vi "Test Pass if in Map.vi"(8 "error in (no error)":errorcluster, 11 "Dummy In":refnum<class "Example Test Case.lvclass">) -> (0 "error out":errorcluster, 3 "Dummy Out":refnum<class "Example Test Case.lvclass">)   [LabVIEW 2020, in "Example Test Case.lvclass"]
doc: "Failing test"
uses:
  Example Test Case.lvclass
  C:/git/astemes-lunit/source/API/LUnit Test Case/LUnit Test Case.lvclass
  API/LUnit Test Case/LUnit Test Case.lvclass/LUnit Test Case.ctl
  f7599997-06c6-4163-a399-60519fa8dddf.vi
  API/LUnit Test Case/Assertions/Pass If.vi
  API/LUnit Test Case/Private/Append Fail Result.vi
  API/LUnit Test Case/Private/Append Pass Result.vi
  API/LUnit Test Case/Private/Run In UI.vi
  <vilib>/Utility/error.llb/Clear Errors.vi
  Example Test Case.lvclass/Example Test Case.ctl
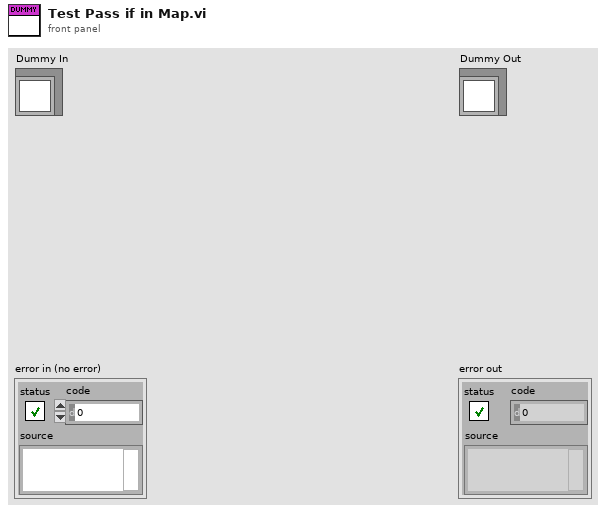
[diagram p1: front panel]
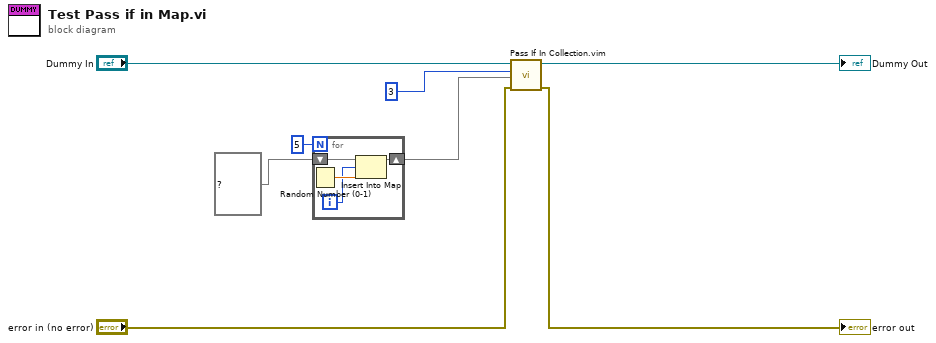
[diagram p0: block diagram]
diagram:
  n1 = for {
    N: 5 -> [_]
    shift-right: [w11] -> w1
    shift-left: map{i32, dbl} {} ("map") -> [w12]
    i -> [w9]
    n2 = Random Number (0-1)() -> (number: 0 to 1=w10:dbl)
    n3 = Insert Into Map(map in=w12, key=w9, value=w10) -> (map out=w11:map{i32, dbl})  [unwired: 2 out]
  }
  n4 = call "Pass If In Collection.vim"("error in (no error)"="error in (no error)", "Collection"=w1, "Expected Element"=3, "LUnit Test Case In"="Dummy In") -> ("error out"=→"error out":errorcluster, "LUnit Test Case Out"=→"Dummy Out":refnum<class "Example Test Case.lvclass">)  [unwired: 6 in]
